vi "GetData.vi"(8 "File":path=path "10 Ft", 11 "file (use dialog)":path) -> (0 "Acceleration Limit (fps^2)":dbl, 1 "Sample Period (s)":dbl, 2 "Velocity Limit (fps)":dbl, 3 "Trajectory Data":T3(array[cluster]), 4 "Commands":T2(array[cluster]) {"System" items=["Elevator", "Floating Intake", "Carriage Intake"]; "System Selection" items=["Elevator", "Floating Intake", "Carriage Intake"]}, 5 "Points":cluster{"x":dbl, "y":dbl, "th":dbl}[](array[cluster]), 6 "Description":string, 7 "Cluster":cluster{"Time (s)":dbl, "Distance (ft)":dbl})   [LabVIEW 2018]
doc: "Getting trajectory data from the roboRio"
uses:
  Availible Command systems for auto.ctl
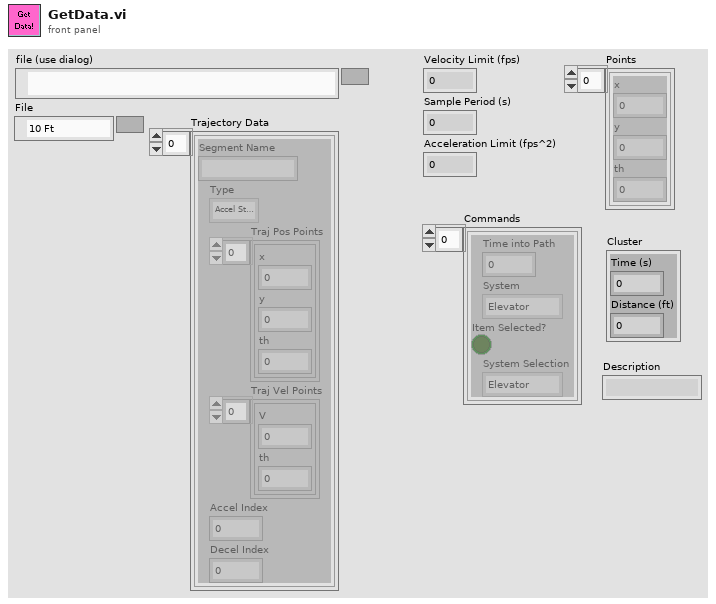
[diagram p1: front panel]
types:
  T1 = typedef "Availible Command systems for auto.ctl" = u16
  T2 = cluster{"Time into Path":dbl, "System":T1, "Item Selected?":bool, "System Selection":T1}[]
  T3 = cluster{"Segment Name":string, "Type":enum16{"Accel Straight", "Const Straight", "Blend", "Circle"}, "Traj Pos Points":cluster{"x":dbl, "y":dbl, "th":dbl}[], "Traj Vel Points":cluster{"V":dbl, "th":dbl}[], "Accel Index":i32, "Decel Index":i32}[]
  T4 = cluster{"Sample Period (s)":dbl, "Limits":cluster{"Velocity (fps)":dbl, "Acceleration (fps^2)":dbl, "Jerk (fps^3)":dbl}, "Conditions":cluster{"vInitial (fps)":dbl, "vFinal (fps)":dbl}}
  T5 = cluster{"Velocity Limit (fps)":dbl, "Sample Period (s)":dbl, "Acceleration Limit (fps^2)":dbl}
  T6 = cluster{"Sample Period (s)":dbl, "Limits":cluster{"Velocity (fps)":dbl, "Acceleration (fps^2)":dbl, "Jerk (fps^3)":dbl}, "Conditions":cluster{"vInitial (fps)":dbl, "vFinal (fps)":dbl}, "Min Rads":dbl[]}
  T7 = cluster{"Sample Period (s)":dbl, "Limits":cluster{"Velocity (fps)":dbl, "Acceleration (fps^2)":dbl, "Jerk (fps^3)":dbl}, "Conditions":cluster{"vInitial (fps)":dbl, "vFinal (fps)":dbl}, "Angular Accelerations":cluster{"Angular \nAccelerations":dbl[], "Override Limits?":bool[]}}
  T8 = cluster{"Time into Path":dbl, "System":u16, "Item Selected?":bool, "System Selection":u16}[]
  T9 = cluster{"Velocity (fps)":dbl, "Acceleration (fps^2)":dbl, "Jerk (fps^3)":dbl}
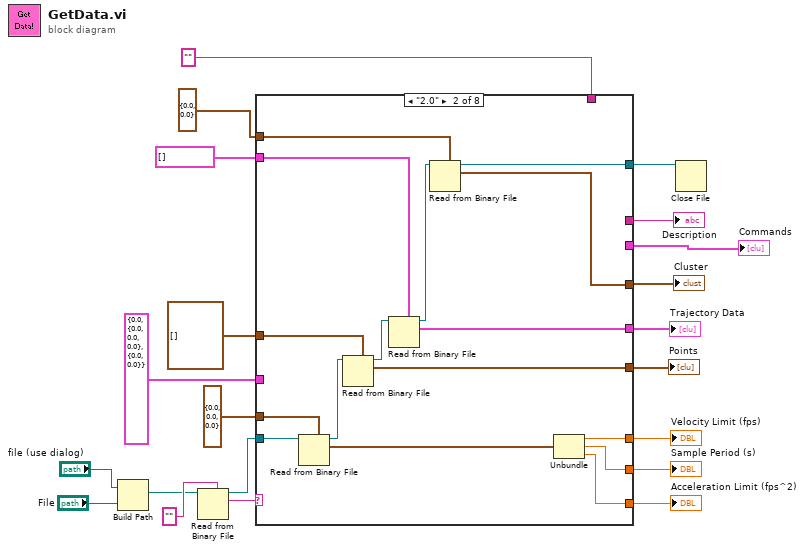
[diagram p0: block diagram]
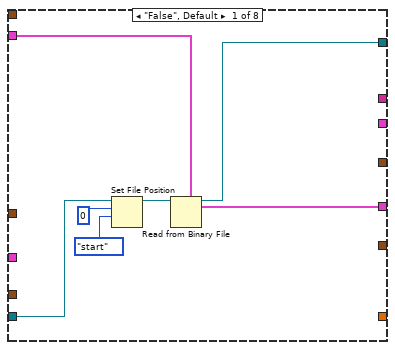
[diagram p2: hidden frame]
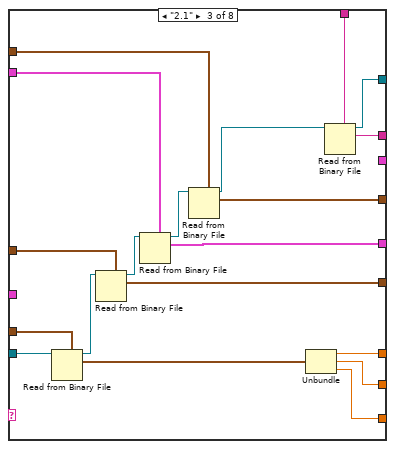
[diagram p3: hidden frame]
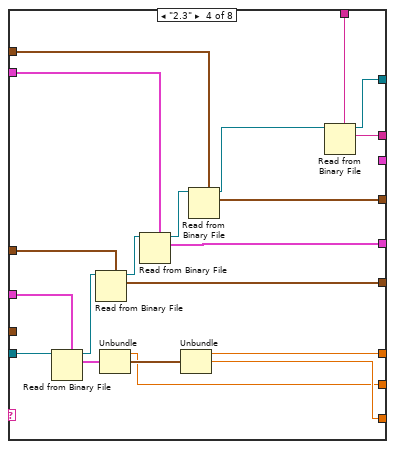
[diagram p4: hidden frame]
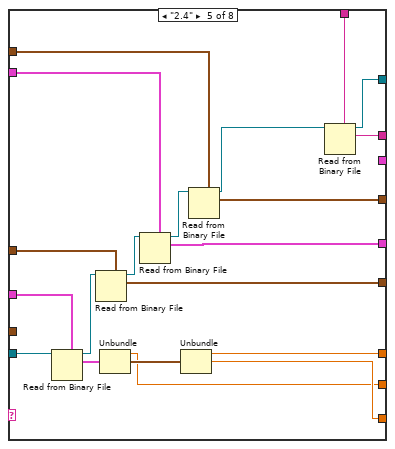
[diagram p5: hidden frame]
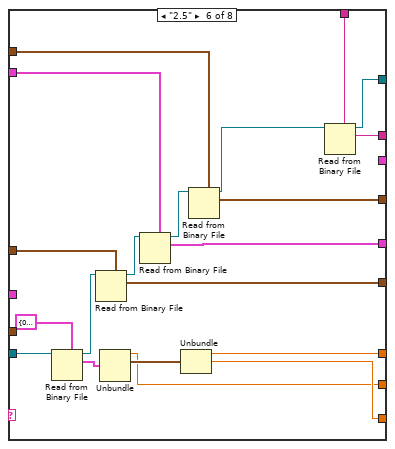
[diagram p6: hidden frame]
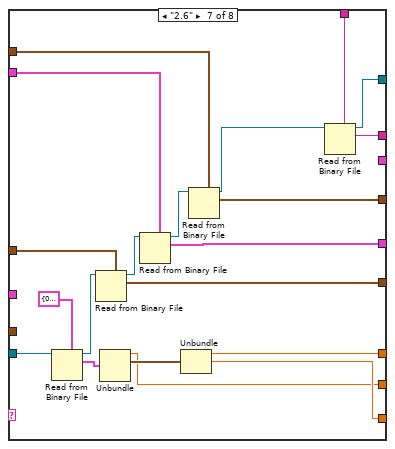
[diagram p7: hidden frame]
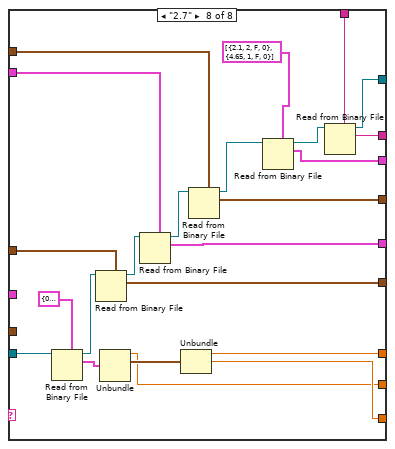
[diagram p8: hidden frame]
diagram:
  n1 = Build Path(base path="file (use dialog)", name or relative path="File") -> (appended path=w4:path)
  n2 = Read from Binary File(5:"", 11:w4) -> (2:w20:string, 3:w19:refnum<file>)  [unwired: 4 in, 2 out]
  n3 = case shown="\"2.0\"" w20 {
    tunnel: w19 -> [w23 w43 w62 w82 w102 w122 w142 w165]
    tunnel: T5 {"Velocity Limit (fps)"=0.0, "Sample Period (s)"=0.0, "Acceleration Limit (fps^2)"=0.0} -> [_ w42 w61 _ _ _ _ _]
    tunnel: cluster{"x":dbl, "y":dbl, "th":dbl}[] [] ("Points") -> [_ w40 w59 w80 w100 w120 w140 w163]
    tunnel: [_ w39 w58 w79 w99 w119 w139 w162] -> w10
    tunnel: T3 [] ("Trajectory Data") -> [w25 w38 w57 w78 w98 w118 w138 w161]
    tunnel: [w24 w36 w55 w76 w96 w116 w136 w159] -> w9
    tunnel: cluster{"Time (s)":dbl, "Distance (ft)":dbl} {"Time (s)"=0.0, "Distance (ft)"=0.0} -> [_ w35 w54 w75 w95 w115 w135 w158]
    tunnel: [_ w33 w52 w73 w93 w113 w133 w156] -> w8
    tunnel: [w22 w32 w47 w71 w91 w111 w131 w155] -> w17
    tunnel: [_ w31 w51 w66 w86 w107 w127 w151] -> w13
    tunnel: [_ w30 w50 w64 w84 w105 w125 w149] -> w12
    tunnel: [_ w29 w49 w65 w85 w106 w126 w150] -> w11
    tunnel: "" -> [_ _ w46 w70 w90 w110 w130 w154]
    tunnel: [_ _ w45 w69 w89 w109 w129 w153] -> w6
    tunnel: T4 {"Sample Period (s)"=0.0, "Limits"={"Velocity (fps)"=0.0, "Acceleration (fps^2)"=0.0, "Jerk (fps^3)"=0.0}, "Conditions"={"vInitial (fps)"=0.0, "vFinal (fps)"=0.0}} -> [_ _ _ w68 w88 _ _ _]
    tunnel: [_ _ _ _ _ _ _ w145] -> w1
    frame "False", Default {
      n4 = Set File Position(offset (in bytes) (0)=i64 0, refnum=w23, from (0:start)=enum16{"start", "end", "current"}."start") -> (refnum out=w26:refnum<file>)  [unwired: 1 in, 1 out]
      n5 = Read from Binary File(5:w25, 11:w26) -> (2:w24:T3, 3:w22:refnum<file>)  [unwired: 4 in, 2 out]
    }
    frame "2.0" {
      n6 = Read from Binary File(5:w42, 11:w43) -> (2:w44:T5, 3:w41:refnum<file>)  [unwired: 4 in, 2 out]
      n7 = Read from Binary File(5:w40, 11:w41) -> (2:w39:cluster{"x":dbl, "y":dbl, "th":dbl}[], 3:w37:refnum<file>)  [unwired: 4 in, 2 out]
      n8 = Read from Binary File(5:w38, 11:w37) -> (2:w36:T3, 3:w34:refnum<file>)  [unwired: 4 in, 2 out]
      n9 = Read from Binary File(5:w35, 11:w34) -> (2:w33:cluster{"Time (s)":dbl, "Distance (ft)":dbl}, 3:w32:refnum<file>)  [unwired: 4 in, 2 out]
      n10 = Unbundle(w44) -> ("Velocity Limit (fps)"=w31:dbl, "Sample Period (s)"=w30:dbl, "Acceleration Limit (fps^2)"=w29:dbl)
    }
    frame "2.1" {
      n11 = Read from Binary File(5:w61, 11:w62) -> (2:w63:T5, 3:w60:refnum<file>)  [unwired: 4 in, 2 out]
      n12 = Read from Binary File(5:w59, 11:w60) -> (2:w58:cluster{"x":dbl, "y":dbl, "th":dbl}[], 3:w56:refnum<file>)  [unwired: 4 in, 2 out]
      n13 = Read from Binary File(5:w57, 11:w56) -> (2:w55:T3, 3:w53:refnum<file>)  [unwired: 4 in, 2 out]
      n14 = Read from Binary File(5:w54, 11:w53) -> (2:w52:cluster{"Time (s)":dbl, "Distance (ft)":dbl}, 3:w48:refnum<file>)  [unwired: 4 in, 2 out]
      n15 = Unbundle(w63) -> ("Velocity Limit (fps)"=w51:dbl, "Sample Period (s)"=w50:dbl, "Acceleration Limit (fps^2)"=w49:dbl)
      n16 = Read from Binary File(5:w46, 11:w48) -> (2:w45:string, 3:w47:refnum<file>)  [unwired: 4 in, 2 out]
    }
    frame "2.3" {
      n17 = Read from Binary File(5:w68, 11:w82) -> (2:w83:T4, 3:w81:refnum<file>)  [unwired: 4 in, 2 out]
      n18 = Read from Binary File(5:w80, 11:w81) -> (2:w79:cluster{"x":dbl, "y":dbl, "th":dbl}[], 3:w77:refnum<file>)  [unwired: 4 in, 2 out]
      n19 = Unbundle(w83) -> ("Sample Period (s)"=w64:dbl, "Limits"=w67:T9)  [unwired: 1 out]
      n20 = Read from Binary File(5:w78, 11:w77) -> (2:w76:T3, 3:w74:refnum<file>)  [unwired: 4 in, 2 out]
      n21 = Unbundle(w67) -> ("Velocity (fps)"=w66:dbl, "Acceleration (fps^2)"=w65:dbl)  [unwired: 1 out]
      n22 = Read from Binary File(5:w75, 11:w74) -> (2:w73:cluster{"Time (s)":dbl, "Distance (ft)":dbl}, 3:w72:refnum<file>)  [unwired: 4 in, 2 out]
      n23 = Read from Binary File(5:w70, 11:w72) -> (2:w69:string, 3:w71:refnum<file>)  [unwired: 4 in, 2 out]
    }
    frame "2.4" {
      n24 = Read from Binary File(5:w88, 11:w102) -> (2:w103:T4, 3:w101:refnum<file>)  [unwired: 4 in, 2 out]
      n25 = Read from Binary File(5:w100, 11:w101) -> (2:w99:cluster{"x":dbl, "y":dbl, "th":dbl}[], 3:w97:refnum<file>)  [unwired: 4 in, 2 out]
      n26 = Unbundle(w103) -> ("Sample Period (s)"=w84:dbl, "Limits"=w87:T9)  [unwired: 1 out]
      n27 = Read from Binary File(5:w98, 11:w97) -> (2:w96:T3, 3:w94:refnum<file>)  [unwired: 4 in, 2 out]
      n28 = Unbundle(w87) -> ("Velocity (fps)"=w86:dbl, "Acceleration (fps^2)"=w85:dbl)  [unwired: 1 out]
      n29 = Read from Binary File(5:w95, 11:w94) -> (2:w93:cluster{"Time (s)":dbl, "Distance (ft)":dbl}, 3:w92:refnum<file>)  [unwired: 4 in, 2 out]
      n30 = Read from Binary File(5:w90, 11:w92) -> (2:w89:string, 3:w91:refnum<file>)  [unwired: 4 in, 2 out]
    }
    frame "2.5" {
      n31 = Read from Binary File(5:T6 {"Sample Period (s)"=0.0, "Limits"={"Velocity (fps)"=0.0, "Acceleration (fps^2)"=0.0, "Jerk (fps^3)"=0.0}, "Conditions"={"vInitial (fps)"=0.0, "vFinal (fps)"=0.0}, "Min Rads"=[20.0, 20.0, 20.0, 20.0, 20.0]}, 11:w122) -> (2:w123:T6, 3:w121:refnum<file>)  [unwired: 4 in, 2 out]
      n32 = Read from Binary File(5:w120, 11:w121) -> (2:w119:cluster{"x":dbl, "y":dbl, "th":dbl}[], 3:w117:refnum<file>)  [unwired: 4 in, 2 out]
      n33 = Unbundle(w123) -> ("Sample Period (s)"=w105:dbl, "Limits"=w108:T9)  [unwired: 2 out]
      n34 = Read from Binary File(5:w118, 11:w117) -> (2:w116:T3, 3:w114:refnum<file>)  [unwired: 4 in, 2 out]
      n35 = Unbundle(w108) -> ("Velocity (fps)"=w107:dbl, "Acceleration (fps^2)"=w106:dbl)  [unwired: 1 out]
      n36 = Read from Binary File(5:w115, 11:w114) -> (2:w113:cluster{"Time (s)":dbl, "Distance (ft)":dbl}, 3:w112:refnum<file>)  [unwired: 4 in, 2 out]
      n37 = Read from Binary File(5:w110, 11:w112) -> (2:w109:string, 3:w111:refnum<file>)  [unwired: 4 in, 2 out]
    }
    frame "2.6" {
      n38 = Read from Binary File(5:T7 {"Sample Period (s)"=0.0, "Limits"={"Velocity (fps)"=0.0, "Acceleration (fps^2)"=0.0, "Jerk (fps^3)"=0.0}, "Conditions"={"vInitial (fps)"=0.0, "vFinal (fps)"=0.0}, "Angular Accelerations"={"Angular \nAccelerations"=[], "Override Limits?"=[]}}, 11:w142) -> (2:w143:T7, 3:w141:refnum<file>)  [unwired: 4 in, 2 out]
      n39 = Read from Binary File(5:w140, 11:w141) -> (2:w139:cluster{"x":dbl, "y":dbl, "th":dbl}[], 3:w137:refnum<file>)  [unwired: 4 in, 2 out]
      n40 = Unbundle(w143) -> ("Sample Period (s)"=w125:dbl, "Limits"=w128:T9)  [unwired: 2 out]
      n41 = Read from Binary File(5:w138, 11:w137) -> (2:w136:T3, 3:w134:refnum<file>)  [unwired: 4 in, 2 out]
      n42 = Unbundle(w128) -> ("Velocity (fps)"=w127:dbl, "Acceleration (fps^2)"=w126:dbl)  [unwired: 1 out]
      n43 = Read from Binary File(5:w135, 11:w134) -> (2:w133:cluster{"Time (s)":dbl, "Distance (ft)":dbl}, 3:w132:refnum<file>)  [unwired: 4 in, 2 out]
      n44 = Read from Binary File(5:w130, 11:w132) -> (2:w129:string, 3:w131:refnum<file>)  [unwired: 4 in, 2 out]
    }
    frame "2.7" {
      n45 = Read from Binary File(5:T7 {"Sample Period (s)"=0.0, "Limits"={"Velocity (fps)"=0.0, "Acceleration (fps^2)"=0.0, "Jerk (fps^3)"=0.0}, "Conditions"={"vInitial (fps)"=0.0, "vFinal (fps)"=0.0}, "Angular Accelerations"={"Angular \nAccelerations"=[], "Override Limits?"=[]}}, 11:w165) -> (2:w166:T7, 3:w164:refnum<file>)  [unwired: 4 in, 2 out]
      n46 = Read from Binary File(5:w163, 11:w164) -> (2:w162:cluster{"x":dbl, "y":dbl, "th":dbl}[], 3:w160:refnum<file>)  [unwired: 4 in, 2 out]
      n47 = Unbundle(w166) -> ("Sample Period (s)"=w149:dbl, "Limits"=w152:T9)  [unwired: 2 out]
      n48 = Read from Binary File(5:w161, 11:w160) -> (2:w159:T3, 3:w157:refnum<file>)  [unwired: 4 in, 2 out]
      n49 = Unbundle(w152) -> ("Velocity (fps)"=w151:dbl, "Acceleration (fps^2)"=w150:dbl)  [unwired: 1 out]
      n50 = Read from Binary File(5:w158, 11:w157) -> (2:w156:cluster{"Time (s)":dbl, "Distance (ft)":dbl}, 3:w147:refnum<file>)  [unwired: 4 in, 2 out]
      n51 = Read from Binary File(5:T8 [{"Time into Path"=2.1, "System"=2, "Item Selected?"=FALSE, "System Selection"=0}, {"Time into Path"=4.65, "System"=1, "Item Selected?"=FALSE, "System Selection"=0}] ("Commands"), 11:w147) -> (2:w145:T8, 3:w146:refnum<file>)  [unwired: 4 in, 2 out]
      n52 = Read from Binary File(5:w154, 11:w146) -> (2:w153:string, 3:w155:refnum<file>)  [unwired: 4 in, 2 out]
    }
  }
  "Velocity Limit (fps)" <- w13
  "Sample Period (s)" <- w12
  "Acceleration Limit (fps^2)" <- w11
  "Points" <- w10
  "Trajectory Data" <- w9
  "Cluster" <- w8
  "Description" <- w6
  "Commands" <- w1
  n53 = Close File(refnum=w17) -> ()  [unwired: 1 in, 2 out]
